vi "Taxi Service.vi"(8 "error in (no error)":errorcluster, 11 "Manejo Turnos in":refnum<class "Manejo Turnos.lvclass">) -> (0 "error out":errorcluster, 3 "Manejo Turnos out":refnum<class "Manejo Turnos.lvclass">)   [LabVIEW 2020, in "Manejo Turnos.lvlib" / "Manejo Turnos.lvclass"]
uses:
  Manejo Turnos.lvclass
  C:/Program Files (x86)/National Instruments/LabVIEW 2020/vi.lib/ActorFramework/Actor/Actor.lvclass
  Manejo Turnos.lvclass/Manejo Turnos.ctl
  <vilib>/ActorFramework/Actor/Actor.lvclass/Actor.ctl
  <vilib>/ActorFramework/Message Enqueuer/Message Enqueuer.lvclass/Message Enqueuer.ctl
  Manejo Turnos Messages/Delete Service Msg/Delete Service Msg.lvclass/Delete Service Msg.ctl
  <vilib>/ActorFramework/Message Enqueuer/Init from Existing Queue.vi
  <vilib>/ActorFramework/Message Enqueuer/Enqueue.vi
  Manejo Turnos Messages/Delete Service Msg/Delete Service Msg.lvclass
  C:/Program Files (x86)/National Instruments/LabVIEW 2020/vi.lib/ActorFramework/Message/Message.lvclass
  <vilib>/ActorFramework/Message Priority Queue/Priority Enqueue.vi
  <vilib>/ActorFramework/Message Enqueuer/Message Enqueuer.lvclass
  <vilib>/ActorFramework/Actor/Actor.lvclass
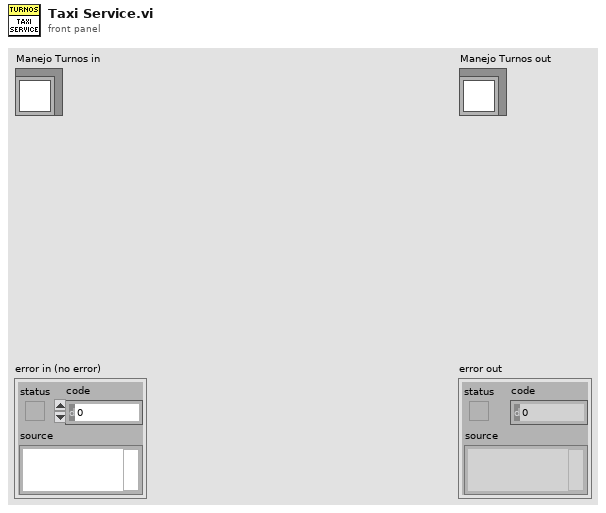
[diagram p1: front panel]
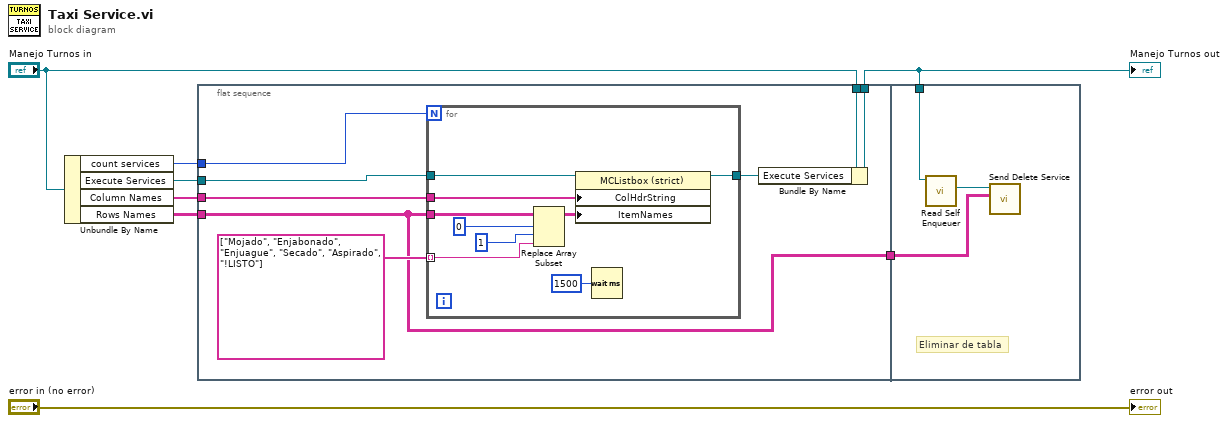
[diagram p0: block diagram]
diagram:
  n1 = Unbundle By Name("Manejo Turnos in") -> ("count services"=w1:i32, "Execute Services"=w7:refnum<vi>, "Column Names"=w6:string[], "Rows Names"=w4:string[][])
  n2 = flat-sequence {
    tunnel: w7 -> [w15]
    tunnel: w6 -> [w14]
    tunnel: [w12] -> w3
    tunnel: "Manejo Turnos in" -> [w11]
    tunnel: w4 -> [w10]
    tunnel: [w10] -> w2
    tunnel: w1 -> [w9]
    tunnel: w3 -> [w28]
    tunnel: w2 -> [w26]
    frame #0 {
      n3 = for {
        N: w9 -> [_]
        tunnel: string[] ["Mojado", "Enjabonado", "Enjuague", "Secado", "Aspirado", "!LISTO"] -> [w17] mode=indexing
        tunnel: w10 -> [w25]
        tunnel: w15 -> [w21]
        tunnel: w14 -> [w20]
        tunnel: [w19] -> w13
        n4 = Replace Array Subset(array=w25, new element=w17, index (row)=0 ("index"), index (col)=1 ("disabled index (col)")) -> (w18:string[][])
        n5 = property class="MCListbox (strict)"(reference=w21, "ColHdrString"=w20, "ItemNames"=w18) -> (reference out=w19:refnum<vi>)  [unwired: 1 in, 1 out]
        n6 = Wait (ms)(milliseconds to wait=u32 1500) -> ()  [unwired: 1 out]
      }
      n7 = Bundle By Name(cluster=w11, "Execute Services"=w13) -> (w12:refnum<class "Manejo Turnos.lvclass">)
    }
    frame #1 {
      # "Eliminar de tabla"
      n8 = call <vilib>:"Read Self Enqueuer.vi"("Actor"=w28) -> ("Self Enqueuer"=w27:refnum<class "Message Enqueuer.lvclass">)  [unwired: 10 in]
      n9 = call "Send Delete Service.vi"("Service Name"=w26, "Message Enqueuer"=w27) -> ()  [unwired: 8 in, 2 out]
    }
  }
  "error out" <- "error in (no error)"
  "Manejo Turnos out" <- w3
